vi "get configuration by alias.vi"(8 "error in":errorcluster, 10 "alias":string, 11 "NISE_CEF_HierarchyRepo in":refnum<class "NISE_CEF_HierarchyRepo.lvclass">) -> (0 "error out":errorcluster, 1 "configuration":refnum<class "NISE_CEF_serializable configuration.lvclass">, 3 "NISE_CEF_HierarchyRepo out":refnum<class "NISE_CEF_HierarchyRepo.lvclass">)   [LabVIEW 2013, in "NISE_CEF_HierarchyRepo.lvclass"]
uses:
  NISE_CEF_HierarchyRepo.lvclass
  serializable configuration/NISE_CEF_serializable configuration.lvclass
  NISE_CEF_HierarchyRepo.lvclass/NISE_CEF_HierarchyRepo.ctl
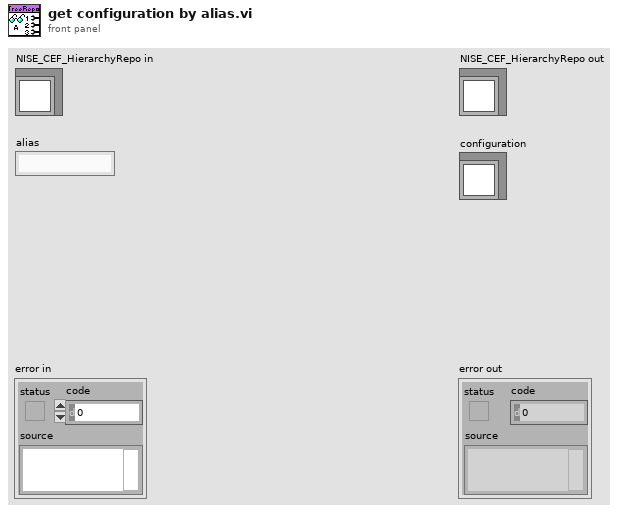
[diagram p1: front panel]
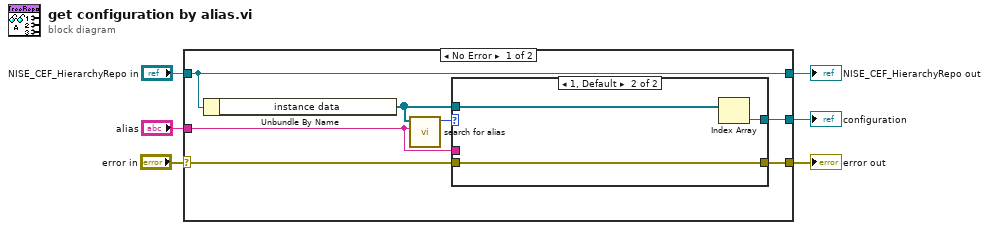
[diagram p0: block diagram]
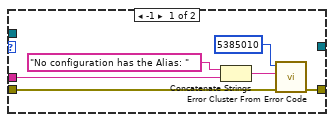
[diagram p2: hidden frame]
diagram:
  n1 = case shown="No Error" "error in" {
    selector: "error in" -> [w9 w24]
    tunnel: [w8 w24] -> w5
    tunnel: [w13 w23] -> w3
    tunnel: "NISE_CEF_HierarchyRepo in" -> [w13 w23]
    tunnel: "alias" -> [w7 _]
    tunnel: [w11 _] -> w1
    frame No Error {
      n2 = Unbundle By Name(w13) -> ("instance data"=w12:refnum<class "NISE_CEF_serializable configuration.lvclass">[])
      n3 = call "search for alias.vi"("alias"=w7, "instance data"=w12) -> ("index"=w10:i32)  [unwired: 9 in]
      n4 = case shown="1, Default" w10 {
        tunnel: w12 -> [_ w22]
        tunnel: [_ w21] -> w11
        tunnel: w9 -> [w19 w20]
        tunnel: [w18 w20] -> w8
        tunnel: w7 -> [w15 _]
        frame -1 {
          n5 = Concatenate Strings("No configuration has the Alias: " ("string"), w15) -> (w16:string)
          n6 = call <vilib>:"Error Cluster From Error Code.vi"("error in (no error)"=w19, "error message (\"\")"=w16, "error code (0)"=5385010) -> ("error out"=w18:errorcluster)  [unwired: 6 in]
        }
        frame 1, Default {
          n7 = Index Array(array=w22) -> (element=w21:refnum<class "NISE_CEF_serializable configuration.lvclass">)  [unwired: 1 in]
        }
      }
    }
    frame Error {
    }
  }
  "error out" <- w5
  "NISE_CEF_HierarchyRepo out" <- w3
  "configuration" <- w1
